vi "Read Sweep Configuration Example.vi"   [LabVIEW 2016, in "SweepControl.lvclass"]
uses:
  SweepControl.lvclass
  Typedefs/Enum - Experiments.ctl
  Typedefs/Continuous B Sweep Configuration--Cluster.ctl
  Typedefs/Enum - Priority.ctl
  Typedefs/Enum - Action.ctl
  Typedefs/Cluster - ScanControl.ctl
  Typedefs/ScanControl.ctl
  Typedefs/Cluster - ScanParamters.ctl
  Typedefs/ScanParamters.ctl
  Typedefs/Sweep Control Configuration--Cluster.ctl
  Transport/Typedefs/Lockin_Sweep Configuration--Cluster.ctl
  Transport/Transport.lvclass
  <userlib>/LevyLab/Krohn Hite 7008/typedefs/Input Configuration-Enum.ctl
  <userlib>/LevyLab/Krohn Hite 7008/Instrument.KH7008.lvclass
  <userlib>/LevyLab/Krohn Hite 7008/typedefs/Shunt-Enum.ctl
  <userlib>/LevyLab/Krohn Hite 7008/typedefs/Gain-Enum.ctl
  <userlib>/LevyLab/Krohn Hite 7008/typedefs/Channel-Enum.ctl
  <userlib>/LevyLab/Krohn Hite 7008/typedefs/KH_control.ctl
  <userlib>/LevyLab/Krohn Hite 7008/typedefs/KH_control_array.ctl
  <userlib>/LevyLab/Lockin-Multichannel/LockinDAQ/Typedefs/REF-cluster.ctl
  <userlib>/LevyLab/Lockin-Multichannel/LockinDAQ/LockinDAQ.lvclass
  <userlib>/LevyLab/Lockin-Multichannel/LockinDAQ/Typedefs/Function-enum.ctl
  <userlib>/LevyLab/Lockin-Multichannel/LockinDAQ/Typedefs/AO-cluster.ctl
  Control Experiment/Typedefs/Wiring Description--cluster.ctl
  Control Experiment/Control Experiment.lvclass
  Control Experiment/Typedefs/Instrument--enum.ctl
  Control Experiment/Typedefs/Experiment Description--cluster.ctl
  <userlib>/_OpenG.lib/dictionary/dictionary.llb/Dictionary Object RefNum - Enum__ogtk.ctl
  <userlib>/_OpenG.lib/dictionary/dictionary.llb/Dictionary Object RefNum__ogtk.ctl
panel:
  # "See block diagram for example of how to use ReadSweepConfigurationFile.vi"
types:
  T1 = typedef "Transport.lvclass/Lockin_Sweep Configuration--Cluster.ctl" = cluster{"Sweep Time (s)":dbl, "Sweep Start (V)":dbl, "Sweep End (V)":dbl, "Sweep Channel":i32}
  T2 = typedef "SweepControl.lvclass/Sweep Control Configuration--Cluster.ctl" = cluster{"Sweep Control":cluster{"Experiment":T3, "Scan parameters":T4, "Scan control":T6}, "Experiment Description":T10, "Wiring Configuration":T13, "Lockin":cluster{"Channels: AO":T14, "Channels: Lockin":T16}, "Krohn Hite":cluster{"Channel Setting":T17}}
  T3 = typedef "SweepControl.lvclass/Enum - Experiments.ctl" = enum16{"IV", "IV_Fast", "IV_Sweep", "Lockin_Vsg", "Lockin_Sweep", "Lockin_Time", "AI WFM time", "Lockin (experimental)"}
  T4 = typedef "SweepControl.lvclass/ScanParamters.ctl" = T5[]
  T5 = typedef "SweepControl.lvclass/Cluster - ScanParamters.ctl" = cluster{"Start":dbl, "End":dbl, "Step":dbl, "Rate":dbl, "wait (ms/mK)":u32, "Address":string, "channel":i32}
  T6 = typedef "SweepControl.lvclass/ScanControl.ctl" = T7[]
  T7 = typedef "SweepControl.lvclass/Cluster - ScanControl.ctl" = cluster{"Priority":T8, "Scan name":T9}
  T8 = typedef "SweepControl.lvclass/Enum - Priority.ctl" = enum16{"Priority 0", "Priority 1", "Priority 2", "Priority 3", "Priority 4", "Priority 5"}
  T9 = typedef "SweepControl.lvclass/Enum - Action.ctl" = enum16{"OFF", "Lockin Amplitude", "Lockin Frequency", "Lockin Bias", "Delay", "Strain", "DAQ Bias", "Magnet Field", "Temperature", "MW f1", "MW f2", "MW Amplitude1", "MW Amplitude2"}
  T10 = typedef "Control Experiment.lvclass/Experiment Description--cluster.ctl" = cluster{"User":string, "Device":string, "Device Path":path, "Device Description":string, "Experiment Path":path, "Experiment Description":string, "Instrument":T11, "Sweep":cluster{"key":string, "value":variant}[], "dictionary":T12}
  T11 = typedef "Control Experiment.lvclass/Instrument--enum.ctl" = enum16{"PPMS", "PPMS2", "DR200", "MNK", "CF900", "MFP3D", "CYPHER", "AGILENT", "JEOL", "THz1", "THz2", "EBL"}
  T12 = typedef "Dictionary Object RefNum__ogtk.ctl" = refnum<k1>
  T13 = typedef "Control Experiment.lvclass/Wiring Description--cluster.ctl" = cluster{"Lockin Ch":i32[], "KH":cluster{"Electrodes":string[], "Labels":string[]}, "not KH":cluster{"Electrodes":string[], "Labels":string[]}}
  T14 = typedef "LockinDAQ.lvclass/AO-cluster.ctl" = cluster{"Ch":i32[], "Amp (V)":dbl[], "DC (V)":dbl[], "f (Hz)":dbl[], "Phase (°)":dbl[], "Function":T15[], "Sweep?":bool[]}
  T15 = typedef "LockinDAQ.lvclass/Function-enum.ctl" = enum16{"Sine", "Triangle", "Square", "Sawtooth"}
  T16 = typedef "LockinDAQ.lvclass/REF-cluster.ctl" = cluster{"Ch":i32[], " f (Hz)":dbl[], "Phase (°)":dbl[], "TC (s)":dbl[], "order":i32[]}
  T17 = typedef "Instrument.KH7008.lvclass/KH_control_array.ctl" = T18[]
  T18 = typedef "Instrument.KH7008.lvclass/KH_control.ctl" = cluster{"Channel":T19, "Gain":T20, "Shunt Resistor":T21, "Input Config":T22}
  T19 = typedef "Instrument.KH7008.lvclass/Channel-Enum.ctl" = enum16{"Channel 1", "Channel 2", "Channel 3", "Channel 4", "Channel 5", "Channel 6", "Channel 7", "Channel 8"}
  T20 = typedef "Instrument.KH7008.lvclass/Gain-Enum.ctl" = enum16{"1x", "10x", "100x", "1000x"}
  T21 = typedef "Instrument.KH7008.lvclass/Shunt-Enum.ctl" = enum16{"Open", "50 Ohms", "500 Ohms", "5k Ohms", "50k Ohms"}
  T22 = typedef "Instrument.KH7008.lvclass/Input Configuration-Enum.ctl" = enum16{"Ground", "SE+ (-gnd)", "SE- (+gnd)", "Differential"}
  T23 = typedef "SweepControl.lvclass/Continuous B Sweep Configuration--Cluster.ctl" = cluster{"Continuous B Sweep":cluster{"Experiment":T3, "B field values":dbl[]}, "Experiment Description":T10, "Wiring Configuration":T13, "Lockin":cluster{"Channels: AO":T14, "Channels: Lockin":T16}, "Krohn Hite":cluster{"Channel Setting":T17}}
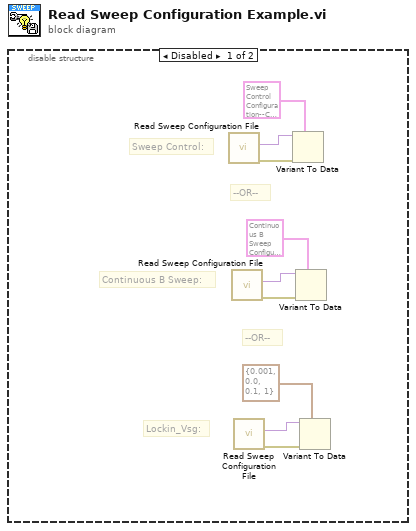
[diagram p0: block diagram]
diagram:
  n1 = disable-structure shown="Disabled" {
    frame Disabled {
      # "Lockin_Vsg:"
      # "Continuous B Sweep:"
      # "Sweep Control:"
      # "--OR--"
      # "--OR--"
      n2 = call "Read Sweep Configuration File.vi"() -> ("error out"=w9:errorcluster, "Data"=w5:variant)  [unwired: 9 in, 1 out]
      n3 = call "Read Sweep Configuration File.vi"() -> ("error out"=w6:errorcluster, "Data"=w4:variant)  [unwired: 9 in, 1 out]
      n4 = call "Read Sweep Configuration File.vi"() -> ("error out"=w8:errorcluster, "Data"=w7:variant)  [unwired: 9 in, 1 out]
      n5 = Variant To Data(error in=w9, type=T2 {"Sweep Control"={"Experiment"=enum."IV", "Scan parameters"=[], "Scan control"=[]}, "Experiment Description"={"User"="", "Device"="", "Device Path"=path "", "Device Description"="", "Experiment Path"=path "", "Experiment Description"="", "Instrument"=enum."PPMS", "Sweep"=[], "dictionary"=refnum}, "Wiring Configuration"={"Lockin Ch"=[], "KH"={"Electrodes"=[], "Labels"=[]}, "not KH"={"Electrodes"=[], "Labels"=[]}}, "Lockin"={"Channels: AO"={"Ch"=[], "Amp (V)"=[], "DC (V)"=[], "f (Hz)"=[], "Phase (°)"=[], "Function"=[], "Sweep?"=[]}, "Channels: Lockin"={"Ch"=[], " f (Hz)"=[], "Phase (°)"=[], "TC (s)"=[], "order"=[]}}, "Krohn Hite"={"Channel Setting"=[]}} ("SweepControl"), Variant=w5) -> ()  [unwired: 2 out]
      n6 = Variant To Data(error in=w6, type=T23 {"Continuous B Sweep"={"Experiment"=enum."IV", "B field values"=[]}, "Experiment Description"={"User"="", "Device"="", "Device Path"=path "", "Device Description"="", "Experiment Path"=path "", "Experiment Description"="", "Instrument"=enum."PPMS", "Sweep"=[], "dictionary"=refnum}, "Wiring Configuration"={"Lockin Ch"=[], "KH"={"Electrodes"=[], "Labels"=[]}, "not KH"={"Electrodes"=[], "Labels"=[]}}, "Lockin"={"Channels: AO"={"Ch"=[], "Amp (V)"=[], "DC (V)"=[], "f (Hz)"=[], "Phase (°)"=[], "Function"=[], "Sweep?"=[]}, "Channels: Lockin"={"Ch"=[], " f (Hz)"=[], "Phase (°)"=[], "TC (s)"=[], "order"=[]}}, "Krohn Hite"={"Channel Setting"=[]}} ("ContinuousBSweep"), Variant=w4) -> ()  [unwired: 2 out]
      n7 = Variant To Data(error in=w8, type=T1 {"Sweep Time (s)"=0.001, "Sweep Start (V)"=0.0, "Sweep End (V)"=0.1, "Sweep Channel"=1} ("LockinVsg Sweep"), Variant=w7) -> ()  [unwired: 2 out]
    }
    frame Enabled {
    }
  }
